vi "Write Message.vi"(8 "error in (no error)":errorcluster, 10 "Message":string, 11 "ConfigDTO in":refnum<class "ConfigDTO.lvclass">) -> (0 "error out":errorcluster, 3 "ConfigDTO out":refnum<class "ConfigDTO.lvclass">)   [LabVIEW 2025, in "DataTransitionObjects.lvlib" / "ConfigDTO.lvclass"]
uses:
  ConfigDTO.lvclass
  ConfigDTO.lvclass/ConfigDTO.ctl
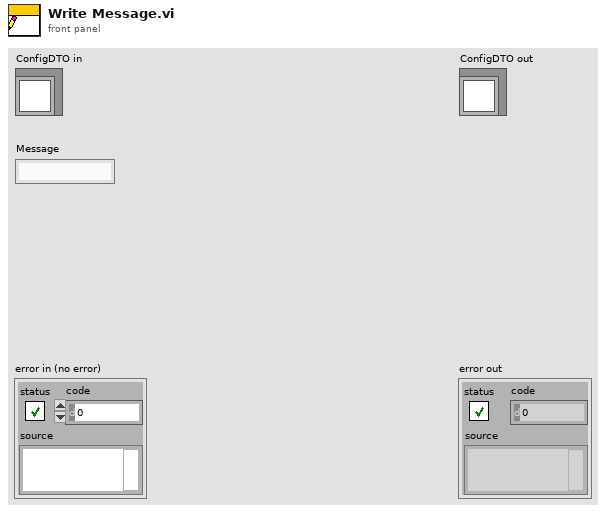
[diagram p1: front panel]
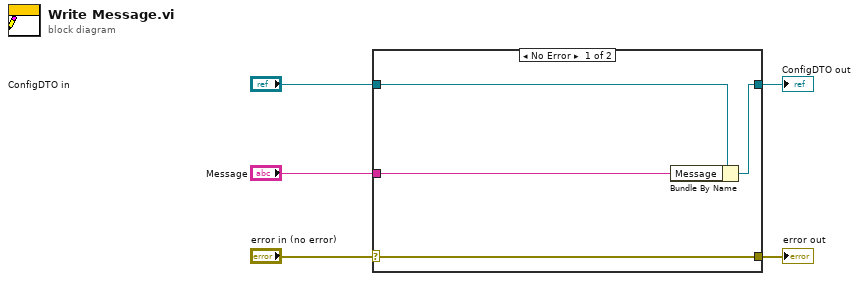
[diagram p0: block diagram]
diagram:
  n1 = case shown="No Error" "error in (no error)" {
    selector: "error in (no error)" -> [w9 w10]
    tunnel: [w9 w10] -> w4
    tunnel: [w7 w11] -> w2
    tunnel: "ConfigDTO in" -> [w8 w11]
    tunnel: "Message" -> [w6 _]
    frame No Error {
      n2 = Bundle By Name(cluster=w8, "Message"=w6) -> (w7:refnum<class "ConfigDTO.lvclass">)
    }
    frame Error {
    }
  }
  "error out" <- w4
  "ConfigDTO out" <- w2
